vi "dataReader.vi"() -> (0 "thetaz":dbl, 1 "thetay":dbl, 2 "thetax":dbl, 3 "平移":cluster{"数值":dbl, "数值 2":dbl, "数值 3":dbl})   [LabVIEW 2012]
uses:
  <vilib>/Utility/file.llb/Read From Spreadsheet File (DBL).vi
panel:
  in  "簇 2":cluster{"数值":dbl, "数值 2":dbl, "数值 3":dbl}
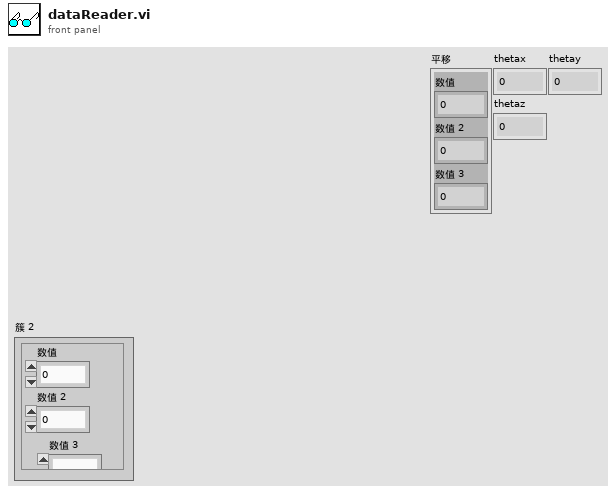
[diagram p1: front panel]
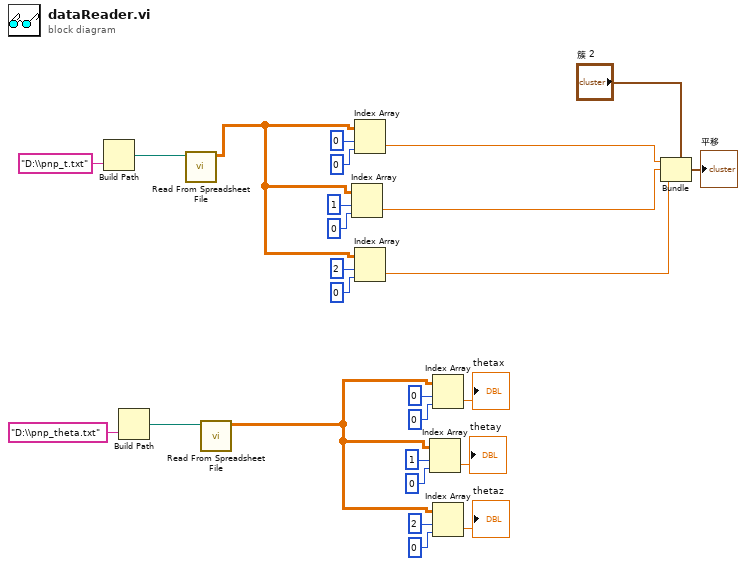
[diagram p0: block diagram]
diagram:
  n1 = Build Path(name or relative path="D:\\pnp_t.txt" ("名称或相对路径")) -> (appended path=w25:path)  [unwired: 1 in]
  n2 = Build Path(name or relative path="D:\\pnp_theta.txt" ("名称或相对路径")) -> (appended path=w23:path)  [unwired: 1 in]
  n3 = call-poly <vilib>:"Read From Spreadsheet File.vi"("file path (dialog if empty)"=w25) -> ("all rows"=w16:dbl[][])  [unwired: 6 in, 4 out]
  n4 = call-poly <vilib>:"Read From Spreadsheet File.vi"("file path (dialog if empty)"=w23) -> ("all rows"=w9:dbl[][])  [unwired: 6 in, 4 out]
  n5 = Index Array(array=w16, index (row)=1 ("禁用的索引 (行)"), index (col)=0 ("禁用的索引 (列)")) -> (element=w3:dbl)
  n6 = Index Array(array=w16, index (row)=0 ("禁用的索引 (行)"), index (col)=0 ("禁用的索引 (列)")) -> (element=w4:dbl)
  n7 = Index Array(array=w16, index (row)=2 ("禁用的索引 (行)"), index (col)=0 ("禁用的索引 (列)")) -> (element=w2:dbl)
  n8 = Index Array(array=w9, index (row)=1 ("禁用的索引 (行)"), index (col)=0 ("禁用的索引 (列)")) -> (element=→"thetay":dbl)
  n9 = Index Array(array=w9, index (row)=0 ("禁用的索引 (行)"), index (col)=0 ("禁用的索引 (列)")) -> (element=→"thetax":dbl)
  n10 = Index Array(array=w9, index (row)=2 ("禁用的索引 (行)"), index (col)=0 ("禁用的索引 (列)")) -> (element=→"thetaz":dbl)
  n11 = Bundle(cluster="簇 2", "数值"=w4, "数值 2"=w3, "数值 3"=w2) -> (→"平移":cluster{"数值":dbl, "数值 2":dbl, "数值 3":dbl})
